vi "CRYReport Pic Update License.vi"   [LabVIEW 2013]
uses:
  <vilib>/registry/registry.llb/Registry RtKey.ctl
  <vilib>/registry/registry.llb/Registry SAM.ctl
  <vilib>/registry/registry.llb/Write Registry Value Simple STR.vi
panel:
  # "Update Register."
types:
  T1 = typedef "Registry SAM.ctl" = enum32{"KEY_QUERY_VALUE", "KEY_SET_VALUE", "KEY_CREATE_SUB_KEY", "KEY_ENUMERATE_SUB_KEYS", "KEY_NOTIFY", "KEY_CREATE_LINK", "KEY_READ", "KEY_WRITE", "KEY_ALL_ACCESS", "KEY_READ | KEY_WRITE"}
  T2 = typedef "Registry RtKey.ctl" = enum32{"HKEY_CLASSES_ROOT", "HKEY_CURRENT_USER", "HKEY_LOCAL_MACHINE", "HKEY_USERS", "HKEY_PERFORMANCE_DATA", "HKEY_CURRENT_CONFIG", "HKEY_DYN_DATA"}
  T3 = typedef "Registry refnum.ctl" = refnum<k1>
  T4 = cluster{"numValues":i32, "maxValueNameLen":i32, "maxValueDataLen":i32}
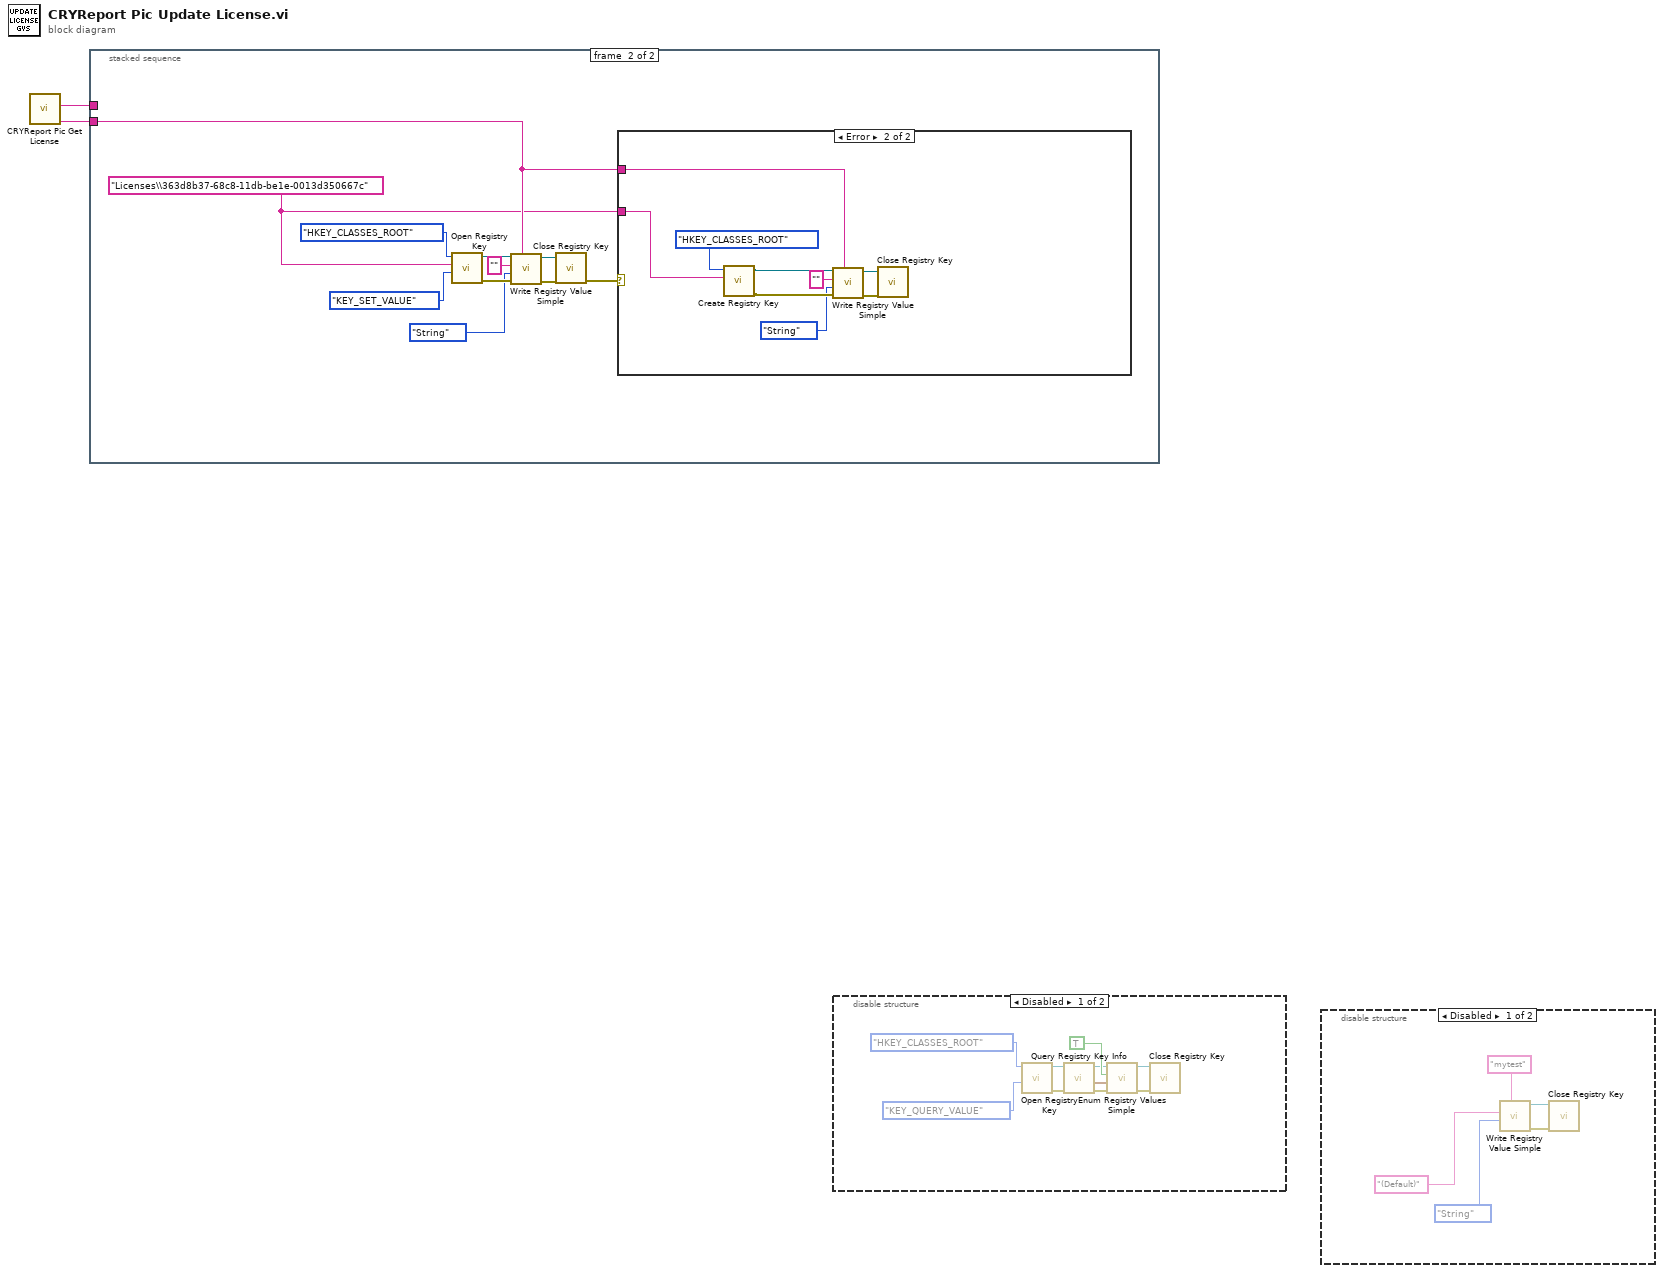
[diagram p0: block diagram]
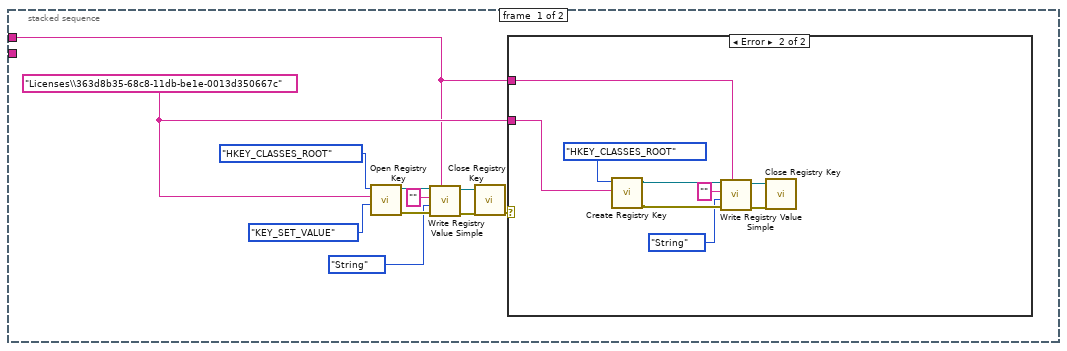
[diagram p2: hidden frame]
diagram:
  n1 = call "CRYReport Pic Get License.vi"() -> ("363d8b37-68c8-11db-be1e-0013d350667c"=w1:string, "363d8b35-68c8-11db-be1e-0013d350667c"=w2:string)  [unwired: 10 in]
  n2 = stacked-sequence {
    tunnel: w2 -> [w3 _]
    tunnel: w1 -> [_ w24]
    frame #0 {
      w6 = "Licenses\\363d8b35-68c8-11db-be1e-0013d350667c" ("subkey")
      n3 = call <vilib>:"Open Registry Key.vi"("security access mask (KEY_READ | KEY_WRITE)"=Registry_SAM."KEY_SET_VALUE", "subkey"=w6, "root key (HKEY_LOCAL_MACHINE)"=Registry_RtKey."HKEY_CLASSES_ROOT") -> ("error out"=w12:errorcluster, "refnum out"=w11:T3)  [unwired: 1 in, 6 out]
      n4 = call-poly <vilib>:"Write Registry Value Simple.vi"("String/Binary data"=w3, "error in (no error)"=w12, "simple data type"=enum16{"String", "Binary", "DWORD"}."String", "value"="", "refnum"=w11) -> ("error out"=w9:errorcluster, "refnum out"=w10:T3)  [unwired: 3 in]
      n5 = call <vilib>:"Close Registry Key.vi"("error in (no error)"=w9, "refnum"=w10) -> ("error out"=w7:errorcluster)  [unwired: 5 out]
      n6 = case shown="Error" w7 {
        tunnel: w6 -> [_ w22]
        tunnel: w3 -> [_ w14]
        frame No Error {
        }
        frame Error {
          n7 = call <vilib>:"Create Registry Key.vi"("subkey"=w22, "root key (HKEY_LOCAL_MACHINE)"=Registry_RtKey."HKEY_CLASSES_ROOT") -> ("error out"=w16:errorcluster, "refnum out"=w17:T3)  [unwired: 7 in, 1 out]
          n8 = call-poly <vilib>:"Write Registry Value Simple.vi"("String/Binary data"=w14, "error in (no error)"=w16, "simple data type"=enum16{"String", "Binary", "DWORD"}."String", "value"="", "refnum"=w17) -> ("error out"=w20:errorcluster, "refnum out"=w19:T3)  [unwired: 3 in]
          n9 = call <vilib>:"Close Registry Key.vi"("error in (no error)"=w20, "refnum"=w19) -> ()  [unwired: 6 out]
        }
      }
    }
    frame #1 {
      w23 = "Licenses\\363d8b37-68c8-11db-be1e-0013d350667c" ("subkey")
      n10 = call <vilib>:"Open Registry Key.vi"("security access mask (KEY_READ | KEY_WRITE)"=Registry_SAM."KEY_SET_VALUE", "subkey"=w23, "root key (HKEY_LOCAL_MACHINE)"=Registry_RtKey."HKEY_CLASSES_ROOT") -> ("error out"=w31:errorcluster, "refnum out"=w30:T3)  [unwired: 1 in, 6 out]
      n11 = call-poly <vilib>:"Write Registry Value Simple.vi"("String/Binary data"=w24, "error in (no error)"=w31, "simple data type"=enum16{"String", "Binary", "DWORD"}."String", "value"="", "refnum"=w30) -> ("error out"=w27:errorcluster, "refnum out"=w28:T3)  [unwired: 3 in]
      n12 = call <vilib>:"Close Registry Key.vi"("error in (no error)"=w27, "refnum"=w28) -> ("error out"=w25:errorcluster)  [unwired: 5 out]
      n13 = case shown="Error" w25 {
        tunnel: w24 -> [_ w35]
        tunnel: w23 -> [_ w34]
        frame No Error {
        }
        frame Error {
          n14 = call <vilib>:"Create Registry Key.vi"("subkey"=w34, "root key (HKEY_LOCAL_MACHINE)"=Registry_RtKey."HKEY_CLASSES_ROOT") -> ("error out"=w37:errorcluster, "refnum out"=w38:T3)  [unwired: 7 in, 1 out]
          n15 = call-poly <vilib>:"Write Registry Value Simple.vi"("String/Binary data"=w35, "error in (no error)"=w37, "simple data type"=enum16{"String", "Binary", "DWORD"}."String", "value"="", "refnum"=w38) -> ("error out"=w41:errorcluster, "refnum out"=w40:T3)  [unwired: 3 in]
          n16 = call <vilib>:"Close Registry Key.vi"("error in (no error)"=w41, "refnum"=w40) -> ()  [unwired: 6 out]
        }
      }
    }
  }
  n17 = disable-structure shown="Disabled" {
    frame Disabled {
      n18 = call <vilib>:"Open Registry Key.vi"("security access mask (KEY_READ | KEY_WRITE)"=Registry_SAM."KEY_QUERY_VALUE", "root key (HKEY_LOCAL_MACHINE)"=Registry_RtKey."HKEY_CLASSES_ROOT") -> ("error out"=w46:errorcluster, "refnum out"=w50:T3)  [unwired: 2 in, 6 out]
      n19 = call <vilib>:"Query Registry Key Info.vi"("error in (no error)"=w46, "refnum"=w50) -> ("error out"=w45:errorcluster, "value info"=w48:T4, "refnum out"=w51:T3)  [unwired: 7 out]
      n20 = call <vilib>:"Enum Registry Values Simple.vi"("error in (no error)"=w45, "value info"=w48, "retrieve data? (F)"=TRUE, "refnum"=w51) -> ("error out"=w44:errorcluster, "refnum out"=w49:T3)  [unwired: 6 out]
      n21 = call <vilib>:"Close Registry Key.vi"("error in (no error)"=w44, "refnum"=w49) -> ()  [unwired: 6 out]
    }
    frame Enabled {
    }
  }
  n22 = disable-structure shown="Disabled" {
    frame Disabled {
      n23 = call-poly <vilib>:"Write Registry Value Simple.vi"("String/Binary data"="mytest", "simple data type"=enum16{"String", "Binary", "DWORD"}."String", "value"="(Default)") -> ("error out"=w54:errorcluster, "refnum out"=w53:T3, "error in (no error)"=w59:errorcluster, "refnum"=w58:T3)  [unwired: 3 in]
      n24 = call <vilib>:"Close Registry Key.vi"("error in (no error)"=w54, "refnum"=w53) -> ()  [unwired: 6 out]
    }
    frame Enabled {
    }
  }
